vi "set.vi"() -> ()   [LabVIEW 2023]
uses:
  Samlink/SAMlink Global Variable.vi
  PFD/PFD_Global.vi
panel:
  out "PFD_HeadingTop":picture
  out "PFD_Heading":picture
  out "PFD_HeadingBack":picture
  out "PFD_AltitudeMid":picture
  out "PFD_AltitudeShort":picture
  out "PFD_Altitude":picture
  out "PFD_Airspeed":picture
  out "PFD_Top":picture
  out "PFD_Attitude":picture
  in  "stop":bool
  out "error out":errorcluster
  in  "PFD Control":T1={"Pitch"=0.0, "Roll"=0.0, "Yaw"=0.0, "Airspeed"=0.0, "Altitude"=0.0, "Ground Altitude"=0.0, "Top Control"={"Arm"=FALSE, "mav_mode"=1, "Mission Mode"=21, "Top Error Ind"={"Batt Stats"={"Active"=TRUE, "State"=FALSE}, "Sat Stats"={"Active"=TRUE, "State"=FALSE}, "Radio Stats"={"Active"=TRUE, "State"=FALSE}, "Sensor Stats"={"Active"=TRUE, "State"=FALSE}}}} {"Yaw" format="%#_13g"}
  in  "VISA resource name":refnum<visa-resource-name>
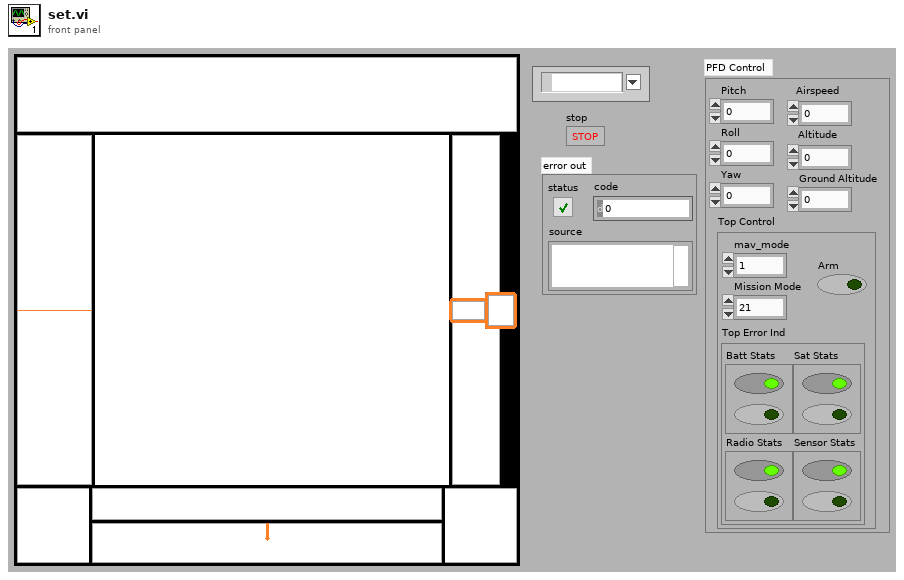
[diagram p1: front panel]
types:
  T1 = cluster{"Pitch":dbl, "Roll":dbl, "Yaw":dbl, "Airspeed":dbl, "Altitude":dbl, "Ground Altitude":dbl, "Top Control":cluster{"Arm":bool, "mav_mode":i16, "Mission Mode":i16, "Top Error Ind":cluster{"Batt Stats":cluster{"Active":bool, "State":bool}, "Sat Stats":cluster{"Active":bool, "State":bool}, "Radio Stats":cluster{"Active":bool, "State":bool}, "Sensor Stats":cluster{"Active":bool, "State":bool}}}}
  T2 = cluster{"color1":u32, "color2":u32, "color_line":u32}
  T3 = cluster{"Air Color":u32, "Line Color":u32, "Ground Color":u32, "Text Color":u32}
  T4 = cluster{"airspeed":sgl, "groundspeed":sgl, "heading":i16, "throttle":u16, "alt (MSL)":sgl, "climb":sgl}
  T5 = cluster{"Timestamp":u32, "roll":sgl, "pitch":sgl, "yaw":sgl, "roll speed deg/s":sgl, "pitch speed deg/s":sgl, "yaw speed deg/s":sgl}
  T6 = cluster{"Heading":dbl, "Alt (m) (MSL)":sgl, "Lon":sgl, "Lat":sgl, "Alt (m) (relativ)":sgl}
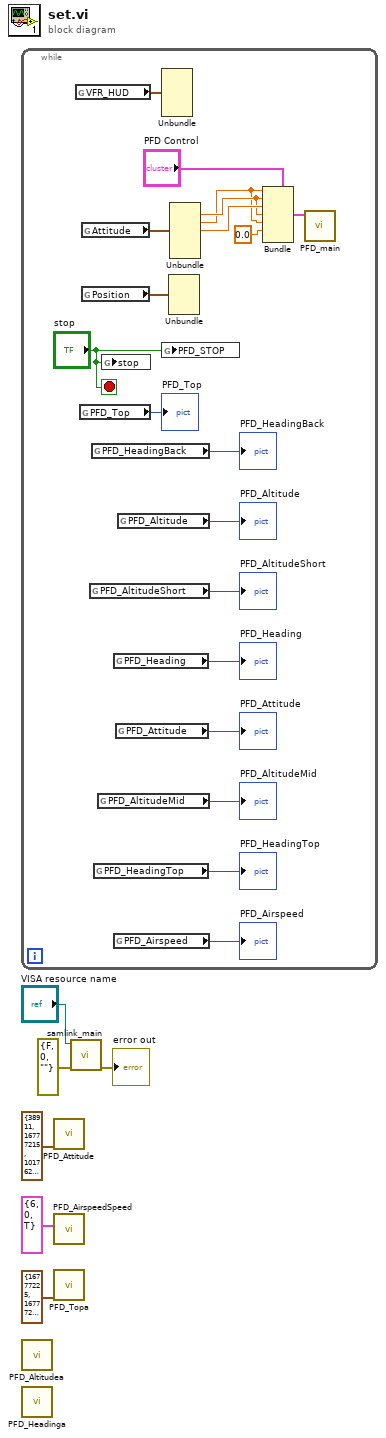
[diagram p0: block diagram]
diagram:
  n1 = while {
    stop <- "stop" stop-if-true
    n2 = global read "SAMlink Global Variable.vi" "VFR_HUD"() -> (w9:T4)
    n3 = global read "PFD_Global.vi" "PFD_Top"() -> (→"PFD_Top":picture)
    n4 = global read "SAMlink Global Variable.vi" "Attitude"() -> (w22:T5)
    n5 = global read "SAMlink Global Variable.vi" "Position"() -> (w20:T6)
    n6 = global read "PFD_Global.vi" "PFD_AltitudeShort"() -> (→"PFD_AltitudeShort":picture)
    n7 = global read "PFD_Global.vi" "PFD_HeadingBack"() -> (→"PFD_HeadingBack":picture)
    n8 = global read "PFD_Global.vi" "PFD_HeadingTop"() -> (→"PFD_HeadingTop":picture)
    n9 = global read "PFD_Global.vi" "PFD_AltitudeMid"() -> (→"PFD_AltitudeMid":picture)
    n10 = global write "SAMlink Global Variable.vi" "stop"("stop") -> ()
    n11 = global read "PFD_Global.vi" "PFD_Heading"() -> (→"PFD_Heading":picture)
    n12 = global read "PFD_Global.vi" "PFD_Airspeed"() -> (→"PFD_Airspeed":picture)
    n13 = global read "PFD_Global.vi" "PFD_Attitude"() -> (→"PFD_Attitude":picture)
    n14 = global read "PFD_Global.vi" "PFD_Altitude"() -> (→"PFD_Altitude":picture)
    n15 = Unbundle(w9) -> ()  [unwired: 6 out]
    n16 = global write "PFD_Global.vi" "PFD_STOP"("stop") -> ()
    n17 = Unbundle(w20) -> ()  [unwired: 5 out]
    n18 = Unbundle(w22) -> ("roll"=w8:sgl, "pitch"=w7:sgl, "yaw"=w21:sgl)  [unwired: 4 out]
    n19 = Bundle(cluster="PFD Control", "Pitch"=w7, "Roll"=w8, "Yaw"=w21, "Airspeed"=w8, "Altitude"=w7, "Ground Altitude"=0.0) -> (w24:T1)  [unwired: 1 in]
    n20 = call "PFD_main.vi"("PFD Control"=w24) -> ()  [unwired: 11 in]
  }
  n21 = call "PFD_Altitudea.vi"() -> ()  [unwired: 9 in, 3 out]
  n22 = call "PFD_Headinga.vi"() -> ()  [unwired: 8 in, 4 out]
  n23 = call "PFD_Attitude.vi"("Color Palette"=T3 {"Air Color"=38911, "Line Color"=16777215, "Ground Color"=10176273, "Text Color"=16777215}) -> ()  [unwired: 9 in, 2 out]
  n24 = call "PFD_AirspeedSpeed.vi"("Airspeedminmax"=cluster{"Max":i16, "Min":i16, "Show":bool} {"Max"=6, "Min"=0, "Show"=TRUE}) -> ()  [unwired: 9 in, 2 out]
  n25 = call "PFD_Topa.vi"("color_palette"=T2 {"color1"=16777225, "color2"=16777224, "color_line"=16777225}) -> ()  [unwired: 9 in, 2 out]
  n26 = call "samlink_main.vi"("error in"=errorcluster {"status"=FALSE, "code"=0, "source"=""}, "VISA resource name"="VISA resource name") -> ("error out"=→"error out":errorcluster)  [unwired: 9 in]
